vi "OpenTalonDrive.vi"   [LabVIEW 2016]
uses:
  <vilib>/Rock Robotics/WPI/ThirdParty/CanMotor/TalonSRX/WPI_CANTalonSRX_APIControlMode.ctl
  <vilib>/Rock Robotics/WPI/SafetyOutput/WPI_SafetyOutputConfigMenu.ctl
  <vilib>/Rock Robotics/WPI/ThirdParty/CanMotor/TalonSRX/WPI_CANTalonSRX_APIFeedbackSelect.ctl
  <vilib>/Rock Robotics/WPI/RobotDrive/WPI_RobotDriveOpen2MotorWithExistingMotors.vi
types:
  T1 = typedef "WPI_CANTalonSRX_APIFeedbackSelect.ctl" = enum16{"Digital Quadrature Encoder", "Analog Potentiometer", "Analog Encoder", "Count on Quad-A (Rising-Edge)", "Count on Quad-A (Falling-Edge)", "CTR Magnetic Enc (Absolute)", "CTR Magnetic Enc (Relative)", "Pulse Width"}
  T2 = typedef "WPI_SafetyOutputConfigMenu.ctl" = enum16{"Enable", "Disable"}
  T3 = typedef "WPI_CANTalonSRX_APIControlMode.ctl" = enum8{"Percent VBus", "Speed", "Position", "Slave", "Unchanged / Invalid", "Voltage Compensation", "Current", "Motion Profile", "Motion Magic"}
  T4 = typedef "WPI_MotorControlDeviceRef.ctl" = cluster{"DeviceStatus":errorcluster, "Type":T5, "PWM":cluster{"PWM Channel":T6, "DeadBand":T7}, "CAN":cluster{"Device Number":u8, "SetOutput VI Ref":variant, "GetOutput VI Ref":variant, "Enable VI Ref":variant, "Disable VI Ref":variant, "Data":variant}, "Invert":bool}
  T5 = typedef "WPI_MotorControlType.ctl" = enum16{"PWM", "CAN"}
  T6 = typedef "FPGA_DIOPWMChannel.ctl" = enum8{"PWM 0", "PWM 1", "PWM 2", "PWM 3", "PWM 4", "PWM 5", "PWM 6", "PWM 7", "PWM 8", "PWM 9", "PWM MXP 0", "PWM MXP 1", "PWM MXP 2", "PWM MXP 3", "PWM MXP 4", "PWM MXP 5", "PWM MXP 6", "PWM MXP 7", "PWM MXP 8", "PWM MXP 9", "Invalid"}
  T7 = typedef "WPI_PWMDeadband.ctl" = cluster{"Name":string, "maxPositivePwm":i32, "minPositivePwm":i32, "centerPwm":i32, "maxNegativePwm":i32, "minNegativePwm":i32, "angularRange":u16}
  T8 = typedef "WPI_RobotDriveDevRef.ctl" = cluster{"DevStatus":errorcluster, "Motors[]":T4[], "Square Inputs":bool, "Max Output":dbl}
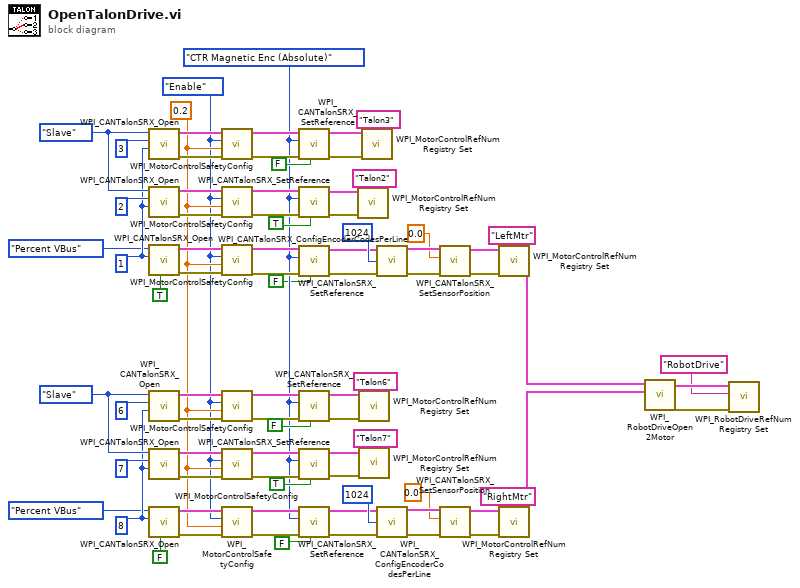
[diagram p0: block diagram]
diagram:
  w19 = WPI_CANTalonSRX_APIFeedbackSelect."CTR Magnetic Enc (Absolute)" ("Feedback Reference")
  w41 = WPI_SafetyOutputConfigMenu."Enable" ("mode")
  w58 = u8 8 ("Device Number")
  w61 = WPI_CANTalonSRX_APIControlMode."Slave" ("Control Mode")
  w42 = 0.2 ("timeout (s)")
  w77 = u8 1 ("Device Number")
  w80 = WPI_CANTalonSRX_APIControlMode."Slave" ("Control Mode")
  n1 = call <vilib>:"WPI_CANTalonSRX_Open.vi"("Master Device Number"=w77, "Device Number"=u8 3, "Control Mode"=w80) -> ("error out"=w72:errorcluster, "CAN Talon SRX Ref"=w73:T4)  [unwired: 7 in]
  n2 = call <vilib>:"WPI_CANTalonSRX_Open.vi"("Master Device Number"=w77, "Device Number"=u8 2, "Control Mode"=w80) -> ("error out"=w70:errorcluster, "CAN Talon SRX Ref"=w71:T4)  [unwired: 7 in]
  n3 = call <vilib>:"WPI_CANTalonSRX_Open.vi"("Invert"=TRUE, "Device Number"=w77, "Control Mode"=WPI_CANTalonSRX_APIControlMode."Percent VBus") -> ("error out"=w74:errorcluster, "CAN Talon SRX Ref"=w75:T4)  [unwired: 7 in]
  n4 = call <vilib>:"WPI_CANTalonSRX_Open.vi"("Master Device Number"=w58, "Device Number"=u8 6, "Control Mode"=w61) -> ("error out"=w53:errorcluster, "CAN Talon SRX Ref"=w54:T4)  [unwired: 7 in]
  n5 = call <vilib>:"WPI_CANTalonSRX_Open.vi"("Master Device Number"=w58, "Device Number"=u8 7, "Control Mode"=w61) -> ("error out"=w51:errorcluster, "CAN Talon SRX Ref"=w52:T4)  [unwired: 7 in]
  n6 = call <vilib>:"WPI_CANTalonSRX_Open.vi"("Invert"=FALSE, "Device Number"=w58, "Control Mode"=WPI_CANTalonSRX_APIControlMode."Percent VBus") -> ("error out"=w55:errorcluster, "CAN Talon SRX Ref"=w56:T4)  [unwired: 7 in]
  n7 = call <vilib>:"WPI_MotorControlSafetyConfig.vi"("error in (no error)"=w72, "timeout (s)"=w42, "mode"=w41, "MotorControlDevRef"=w73) -> ("error out"=w39:errorcluster, "MotorControlDevRef"=w40:T4)  [unwired: 6 in]
  n8 = call <vilib>:"WPI_MotorControlSafetyConfig.vi"("error in (no error)"=w70, "timeout (s)"=w42, "mode"=w41, "MotorControlDevRef"=w71) -> ("error out"=w37:errorcluster, "MotorControlDevRef"=w38:T4)  [unwired: 6 in]
  n9 = call <vilib>:"WPI_MotorControlSafetyConfig.vi"("error in (no error)"=w74, "timeout (s)"=w42, "mode"=w41, "MotorControlDevRef"=w75) -> ("error out"=w22:errorcluster, "MotorControlDevRef"=w23:T4)  [unwired: 6 in]
  n10 = call <vilib>:"WPI_MotorControlSafetyConfig.vi"("error in (no error)"=w53, "timeout (s)"=w42, "mode"=w41, "MotorControlDevRef"=w54) -> ("error out"=w34:errorcluster, "MotorControlDevRef"=w33:T4)  [unwired: 6 in]
  n11 = call <vilib>:"WPI_MotorControlSafetyConfig.vi"("error in (no error)"=w51, "timeout (s)"=w42, "mode"=w41, "MotorControlDevRef"=w52) -> ("error out"=w36:errorcluster, "MotorControlDevRef"=w35:T4)  [unwired: 6 in]
  n12 = call <vilib>:"WPI_MotorControlSafetyConfig.vi"("error in (no error)"=w55, "timeout (s)"=w42, "mode"=w41, "MotorControlDevRef"=w56) -> ("error out"=w26:errorcluster, "MotorControlDevRef"=w27:T4)  [unwired: 6 in]
  n13 = call <vilib>:"WPI_CANTalonSRX_SetReference.vi"("Reverse Closed-Loop Output"=FALSE ("Invert T4"), "error in (no error)"=w39, "Feedback Reference"=w19, "CAN Talon SRX Ref"=w40) -> ("error out"=w5:errorcluster, "CAN Talon SRX Ref"=w4:T4)  [unwired: 6 in]
  n14 = call <vilib>:"WPI_CANTalonSRX_SetReference.vi"("Reverse Closed-Loop Output"=TRUE ("Invert T2"), "error in (no error)"=w37, "Feedback Reference"=w19, "CAN Talon SRX Ref"=w38) -> ("error out"=w7:errorcluster, "CAN Talon SRX Ref"=w6:T4)  [unwired: 6 in]
  n15 = call <vilib>:"WPI_CANTalonSRX_SetReference.vi"("Reverse Closed-Loop Output"=FALSE ("Invert T1"), "error in (no error)"=w22, "Feedback Reference"=w19, "CAN Talon SRX Ref"=w23) -> ("error out"=w20:errorcluster, "CAN Talon SRX Ref"=w21:T4)  [unwired: 6 in]
  n16 = call <vilib>:"WPI_CANTalonSRX_SetReference.vi"("Reverse Closed-Loop Output"=FALSE ("Invert 4"), "error in (no error)"=w34, "Feedback Reference"=w19, "CAN Talon SRX Ref"=w33) -> ("error out"=w9:errorcluster, "CAN Talon SRX Ref"=w8:T4)  [unwired: 6 in]
  n17 = call <vilib>:"WPI_CANTalonSRX_SetReference.vi"("Reverse Closed-Loop Output"=TRUE ("Invert 5"), "error in (no error)"=w36, "Feedback Reference"=w19, "CAN Talon SRX Ref"=w35) -> ("error out"=w12:errorcluster, "CAN Talon SRX Ref"=w11:T4)  [unwired: 6 in]
  n18 = call <vilib>:"WPI_CANTalonSRX_SetReference.vi"("Reverse Closed-Loop Output"=FALSE ("Invert 6"), "error in (no error)"=w26, "Feedback Reference"=w19, "CAN Talon SRX Ref"=w27) -> ("error out"=w24:errorcluster, "CAN Talon SRX Ref"=w25:T4)  [unwired: 6 in]
  n19 = call <vilib>:"WPI_MotorControlRefNum Registry Set.vi"("error in (no error)"=w7, "refnum name"="Talon2", "MotorControlDevRef"=w6) -> ()  [unwired: 7 in, 2 out]
  n20 = call <vilib>:"WPI_MotorControlRefNum Registry Set.vi"("error in (no error)"=w9, "refnum name"="Talon6", "MotorControlDevRef"=w8) -> ()  [unwired: 7 in, 2 out]
  n21 = call <vilib>:"WPI_MotorControlRefNum Registry Set.vi"("error in (no error)"=w12, "refnum name"="Talon7", "MotorControlDevRef"=w11) -> ()  [unwired: 7 in, 2 out]
  n22 = call <vilib>:"WPI_MotorControlRefNum Registry Set.vi"("error in (no error)"=w5, "refnum name"="Talon3", "MotorControlDevRef"=w4) -> ()  [unwired: 7 in, 2 out]
  n23 = call <vilib>:"WPI_CANTalonSRX_ConfigEncoderCodesPerLine.vi"("CAN Talon SRX Ref"=w21, "Number Encoder Lines\n(Counts Per Rotation)"=u32 1024 ("Number Encoder Lines\n(Counts Per Rotation)"), "error in (no error)"=w20) -> ("CAN Talon SRX Ref"=w67:T4, "error out"=w68:errorcluster)  [unwired: 11 in]
  n24 = call <vilib>:"WPI_CANTalonSRX_ConfigEncoderCodesPerLine.vi"("CAN Talon SRX Ref"=w25, "Number Encoder Lines\n(Counts Per Rotation)"=u32 1024 ("Number Encoder Lines\n(Counts Per Rotation)"), "error in (no error)"=w24) -> ("CAN Talon SRX Ref"=w48:T4, "error out"=w49:errorcluster)  [unwired: 11 in]
  n25 = call <vilib>:"WPI_CANTalonSRX_SetSensorPosition.vi"("error in (no error)"=w68, "New Sensor Position"=0.0, "CAN Talon SRX Ref"=w67) -> ("error out"=w65:errorcluster, "CAN Talon SRX Ref"=w64:T4)  [unwired: 7 in]
  n26 = call <vilib>:"WPI_CANTalonSRX_SetSensorPosition.vi"("error in (no error)"=w49, "New Sensor Position"=0.0, "CAN Talon SRX Ref"=w48) -> ("error out"=w46:errorcluster, "CAN Talon SRX Ref"=w45:T4)  [unwired: 7 in]
  n27 = call <vilib>:"WPI_MotorControlRefNum Registry Set.vi"("error in (no error)"=w65, "refnum name"="LeftMtr" ("Ref Name 1"), "MotorControlDevRef"=w64) -> ("MotorControlDevRef"=w17:T4)  [unwired: 7 in, 1 out]
  n28 = call <vilib>:"WPI_MotorControlRefNum Registry Set.vi"("error in (no error)"=w46, "refnum name"="RightMtr" ("Ref Name 2"), "MotorControlDevRef"=w45) -> ("MotorControlDevRef"=w16:T4)  [unwired: 7 in, 1 out]
  n29 = call-poly <vilib>:"WPI_RobotDriveOpen2Motor.vi"("Right Motor Dev Ref"=w16, "Left Motor Dev Ref"=w17) -> ("error out"=w14:errorcluster, "RobotDriveDevRef"=w15:T8)  [unwired: 8 in]
  n30 = call <vilib>:"WPI_RobotDriveRefNum Registry Set.vi"("error in (no error)"=w14, "refnum name"="RobotDrive", "RobotDriveDevRef"=w15) -> ()  [unwired: 7 in, 2 out]
